vi "get typeinfo.vi"(11 "type":T1(ring)=enum."QSFP28") -> (2 "second item names":string[](array[string]), 3 "test items":string[](array[string]))   [LabVIEW 2011]
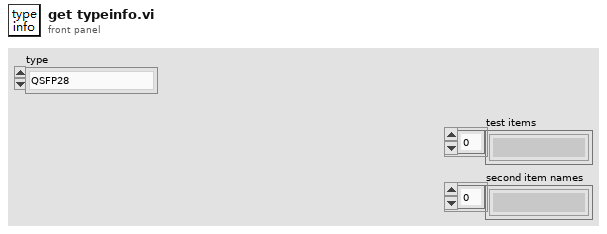
[diagram p1: front panel]
types:
  T1 = enum16{"MINI SAS HD 4X", "MINI SAS 4X", "SFP28", "QSFP28", "SFP+", "SLIM"}
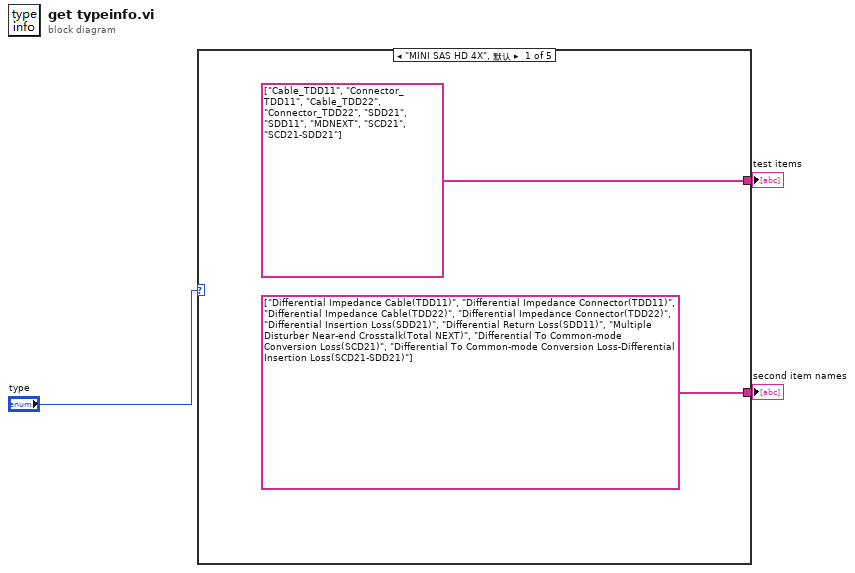
[diagram p0: block diagram]
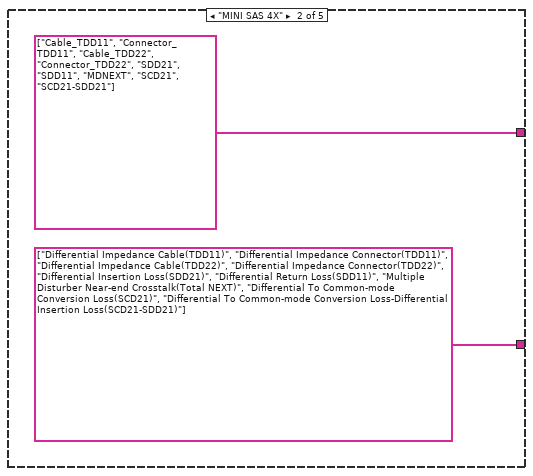
[diagram p2: hidden frame]
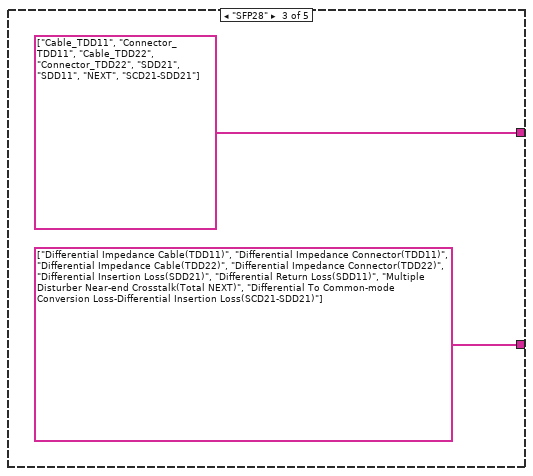
[diagram p3: hidden frame]
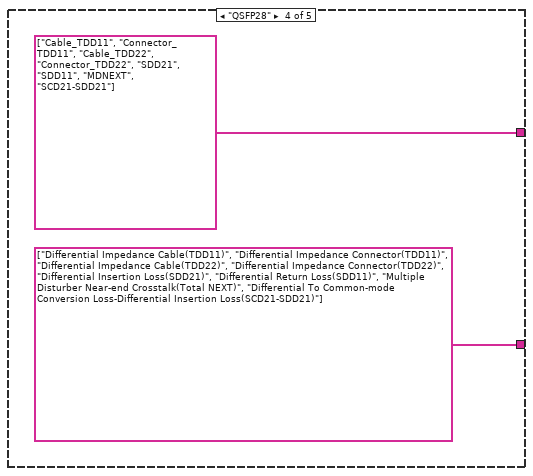
[diagram p4: hidden frame]
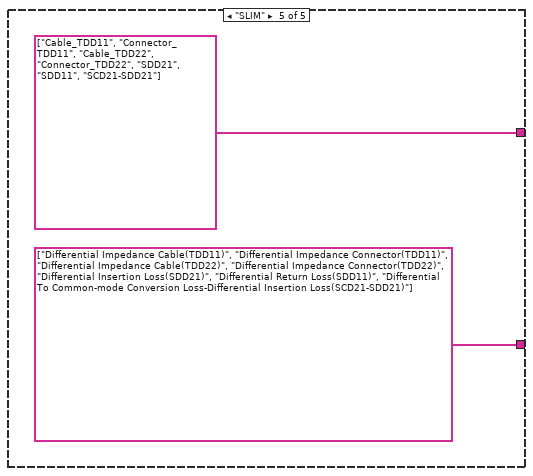
[diagram p5: hidden frame]
diagram:
  n1 = case shown="\"MINI SAS HD 4X\", 默认" "type" {
    tunnel: [string[] ["Cable_TDD11", "Connector_TDD11", "Cable_TDD22", "Connector_TDD22", "SDD21", "SDD11", "MDNEXT", "SCD21", "SCD21-SDD21"] ("test items") string[] ["Cable_TDD11", "Connector_TDD11", "Cable_TDD22", "Connector_TDD22", "SDD21", "SDD11", "MDNEXT", "SCD21", "SCD21-SDD21"] ("test items") string[] ["Cable_TDD11", "Connector_TDD11", "Cable_TDD22", "Connector_TDD22", "SDD21", "SDD11", "NEXT", "SCD21-SDD21"] ("test items") string[] ["Cable_TDD11", "Connector_TDD11", "Cable_TDD22", "Connector_TDD22", "SDD21", "SDD11", "MDNEXT", "SCD21-SDD21"] ("test items") string[] ["Cable_TDD11", "Connector_TDD11", "Cable_TDD22", "Connector_TDD22", "SDD21", "SDD11", "SCD21-SDD21"] ("test items")] -> w3
    tunnel: [string[] ["Differential Impedance Cable(TDD11)", "Differential Impedance Connector(TDD11)", "Differential Impedance Cable(TDD22)", "Differential Impedance Connector(TDD22)", "Differential Insertion Loss(SDD21)", "Differential Return Loss(SDD11)", "Multiple Disturber Near-end Crosstalk(Total NEXT)", "Differential To Common-mode Conversion Loss(SCD21)", "Differential To Common-mode Conversion Loss-Differential Insertion Loss(SCD21-SDD21)"] ("second item names") string[] ["Differential Impedance Cable(TDD11)", "Differential Impedance Connector(TDD11)", "Differential Impedance Cable(TDD22)", "Differential Impedance Connector(TDD22)", "Differential Insertion Loss(SDD21)", "Differential Return Loss(SDD11)", "Multiple Disturber Near-end Crosstalk(Total NEXT)", "Differential To Common-mode Conversion Loss(SCD21)", "Differential To Common-mode Conversion Loss-Differential Insertion Loss(SCD21-SDD21)"] ("second item names") string[] ["Differential Impedance Cable(TDD11)", "Differential Impedance Connector(TDD11)", "Differential Impedance Cable(TDD22)", "Differential Impedance Connector(TDD22)", "Differential Insertion Loss(SDD21)", "Differential Return Loss(SDD11)", "Multiple Disturber Near-end Crosstalk(Total NEXT)", "Differential To Common-mode Conversion Loss-Differential Insertion Loss(SCD21-SDD21)"] ("second item names") string[] ["Differential Impedance Cable(TDD11)", "Differential Impedance Connector(TDD11)", "Differential Impedance Cable(TDD22)", "Differential Impedance Connector(TDD22)", "Differential Insertion Loss(SDD21)", "Differential Return Loss(SDD11)", "Multiple Disturber Near-end Crosstalk(Total NEXT)", "Differential To Common-mode Conversion Loss-Differential Insertion Loss(SCD21-SDD21)"] ("second item names") string[] ["Differential Impedance Cable(TDD11)", "Differential Impedance Connector(TDD11)", "Differential Impedance Cable(TDD22)", "Differential Impedance Connector(TDD22)", "Differential Insertion Loss(SDD21)", "Differential Return Loss(SDD11)", "Differential To Common-mode Conversion Loss-Differential Insertion Loss(SCD21-SDD21)"] ("second item names")] -> w2
    frame "MINI SAS HD 4X", Default {
    }
    frame "MINI SAS 4X" {
    }
    frame "SFP28" {
    }
    frame "QSFP28" {
    }
    frame "SLIM" {
    }
  }
  "test items" <- w3
  "second item names" <- w2
